vi "Test Data Graph01.vi"() -> ()   [LabVIEW 2020]
uses:
  <vilib>/measure/NI_MABase.lvlib
panel:
  in  "文件路径":path=path "C:/Users/26832/Desktop/20230719_134206.tdms"
  in  "Load":bool
  out "XY":cluster{timestamp[], dbl[]}[](graph)
  in  "P1":dbl(slide) scale=3772590125.497653..3772664225.497653 scale format="%<%m/%d %H:%M:%S>T"
  in  "P2":dbl(slide) scale=3772590125.497653..3772664225.497653 scale format="%<%m/%d %H:%M:%S>T"
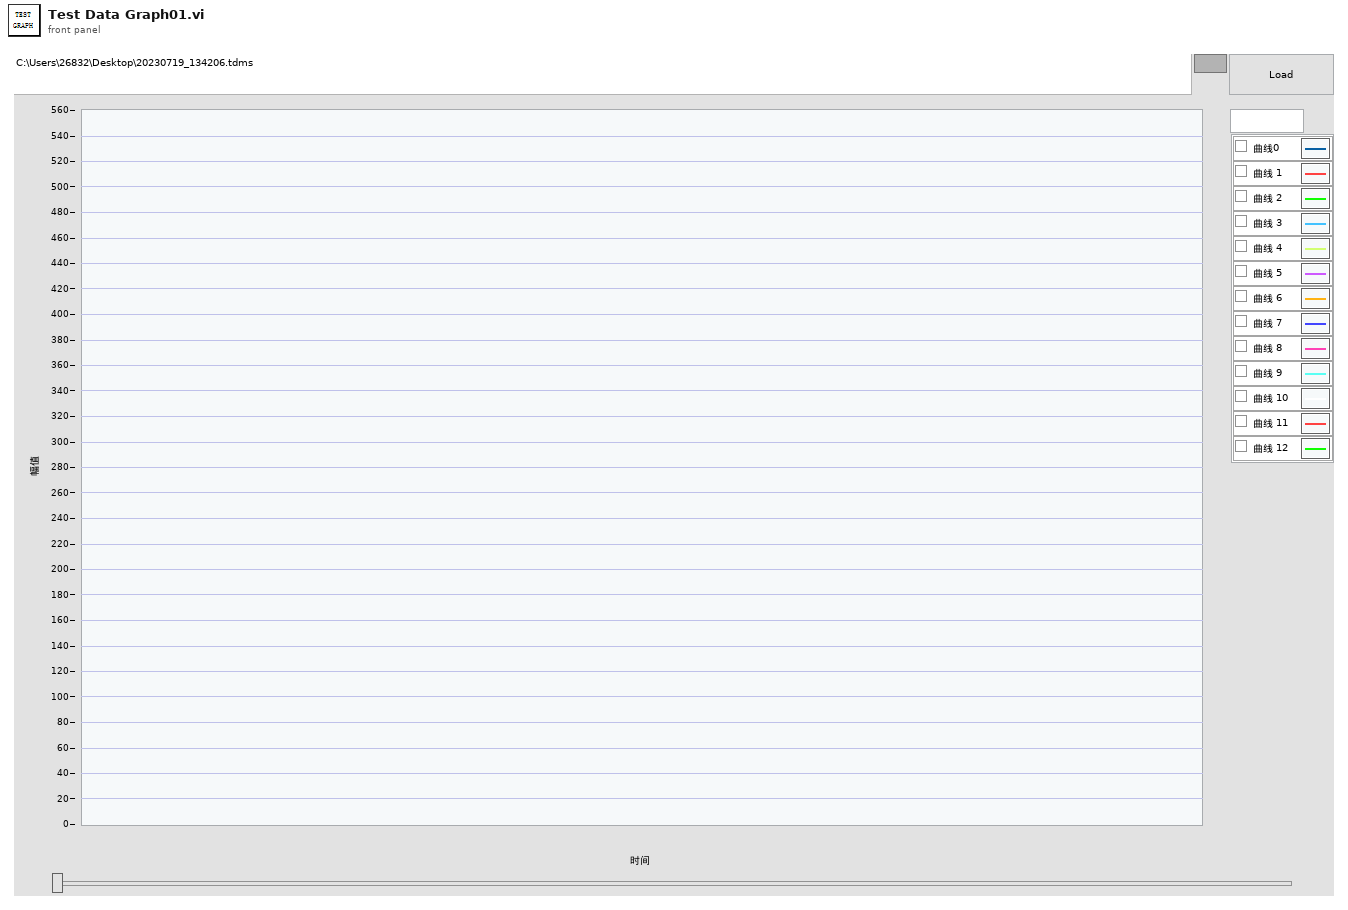
[diagram p1: front panel]
types:
  T1 = cluster{"XY":refnum<vi>, "Maxpoint":i32, "P1":refnum<vi>, "P2":refnum<vi>, "Range":cluster{"IStart":dbl, "CRange":dbl, "IRange":dbl, "CStart":dbl, "Stop":dbl}, "Wave":cluster{"Init":waveform(dbl), "Current":waveform(dbl)}}
  T2 = typedef "LVRangeTypeDef.ctl" = cluster{"Minimum":dbl, "Maximum":dbl, "Increment":dbl, "Minor Increment":dbl, "Start":dbl}
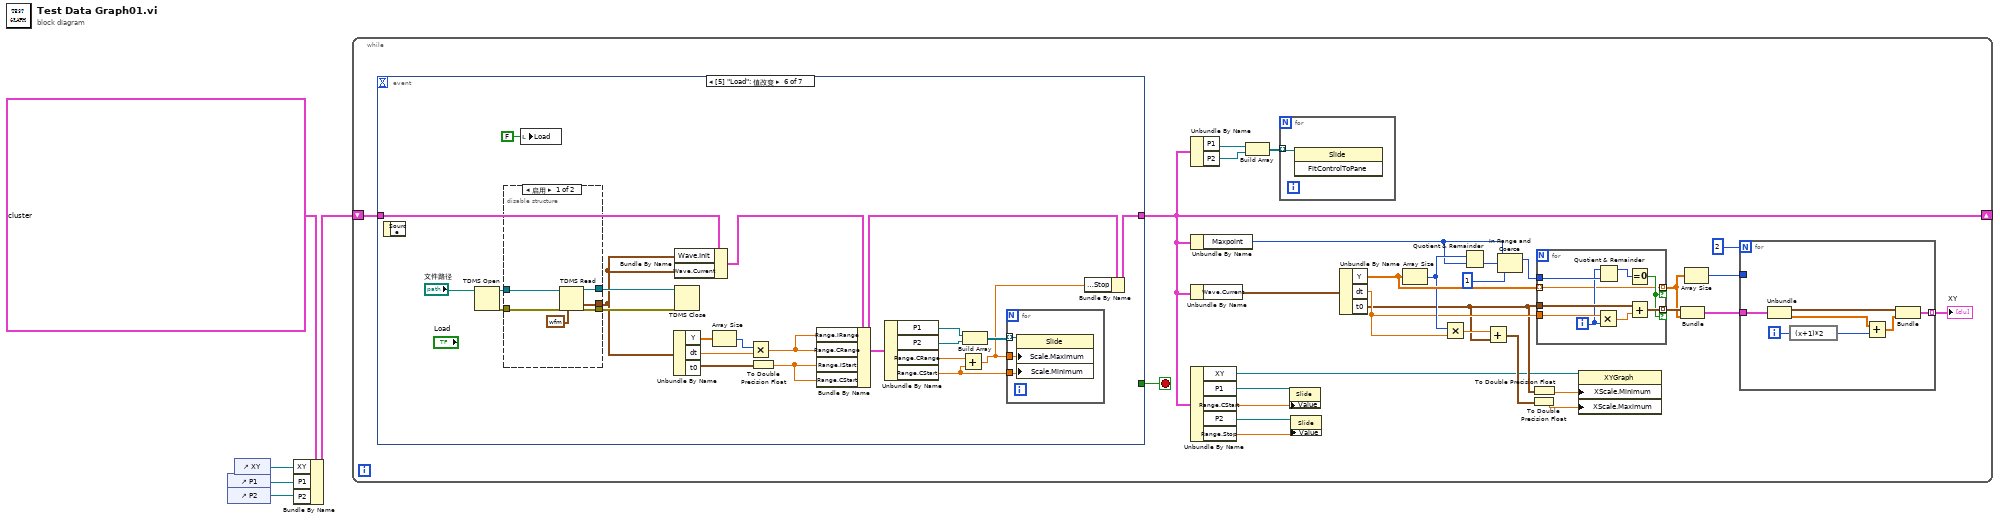
[diagram p0: block diagram]
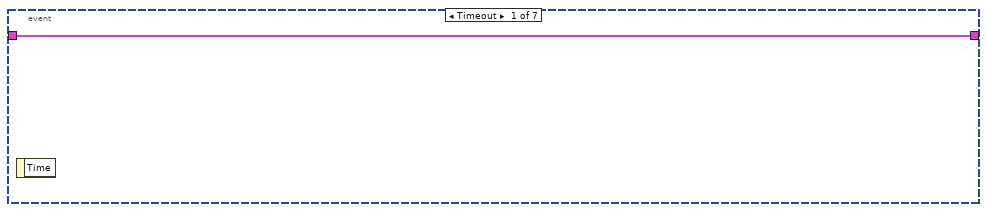
[diagram p2: hidden frame]
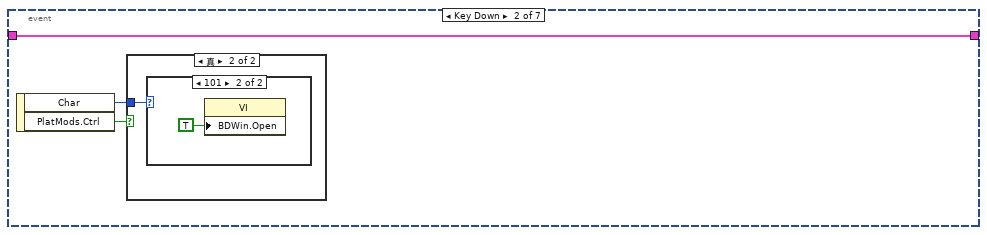
[diagram p3: hidden frame]
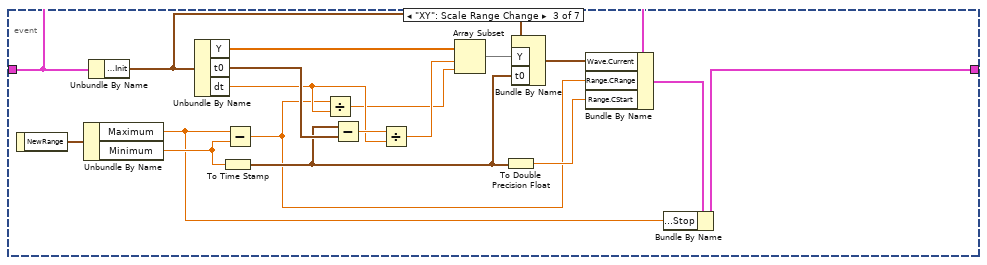
[diagram p6: hidden frame]
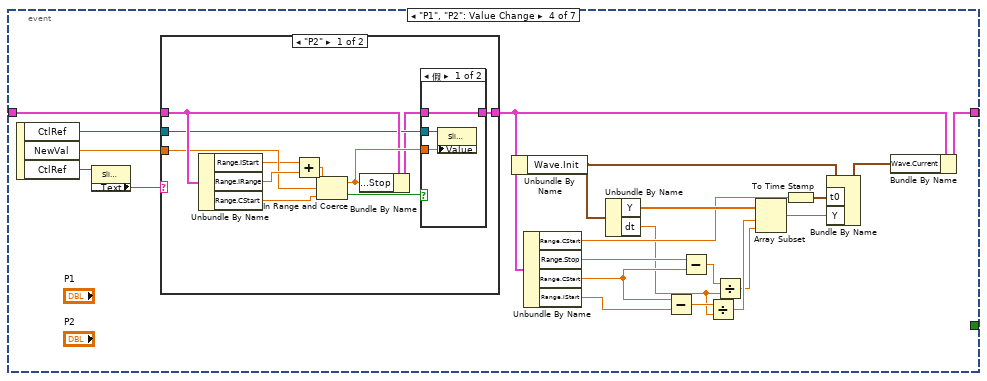
[diagram p7: hidden frame]
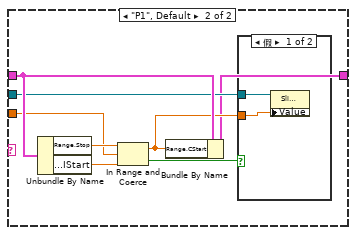
[diagram p9: hidden frame]
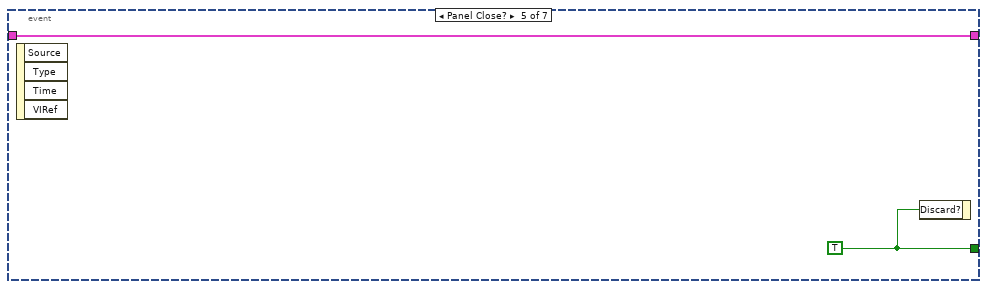
[diagram p11: hidden frame]
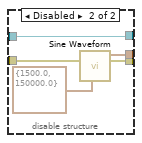
[diagram p12: hidden frame]
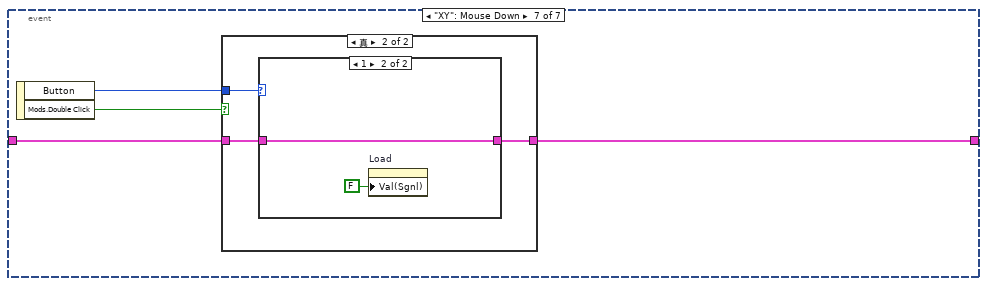
[diagram p13: hidden frame]
diagram:
  n1 = control-ref of="P1"() -> (w2:refnum<vi>)
  n2 = control-ref of="P2"() -> (w1:refnum<vi>)
  n3 = control-ref of="XY"() -> (w3:refnum<vi>)
  n4 = Bundle By Name(cluster=T1 {"XY"=refnum, "Maxpoint"=5000, "P1"=refnum, "P2"=refnum, "Range"={"IStart"=0.0, "CRange"=0.0, "IRange"=0.0, "CStart"=0.0, "Stop"=0.0}, "Wave"={"Init"={"t0"=timestamp(0 s since 1904-01-01), "dt"=1.0, "Y"=[]}, "Current"={"t0"=timestamp(0 s since 1904-01-01), "dt"=1.0, "Y"=[]}}}, "XY"=w3, "P1"=w2, "P2"=w1) -> (w4:T1)
  n5 = while {
    shift-right: [w9] -> _
    shift-left: w4 -> [w34]
    stop <- w35 stop-if-true
    n6 = event shown="[5] \"Load\": 值改变" {
      selector: _ -> [_ _ _ _ _ _ _]
      dyn-events: _ -> [_ _ _ _ _ _ _]
      timeout: _ -> [_ _ _ _ _ _ _]
      tunnel: [_ _ _ _ w124 _ _] -> w35
      tunnel: [w53 w54 w60 w95 w123 w128 w161] -> w9
      tunnel: w34 -> [w53 w54 w67 w97 w123 w142 w162]
      event Timeout {
        n7 = event-data() -> ()  [unwired: 1 in, 1 out]
      }
      event Key Down {
        n8 = event-data() -> ("Char"=w56:i16, "PlatMods.Ctrl"=w55:bool)  [unwired: 1 in]
        n9 = case shown="真" w55 {
          tunnel: w56 -> [_ w57]
          frame False {
          }
          frame True {
            n10 = case shown="101" w57 {
              frame 0, Default {
              }
              frame 101 {
                n11 = property class="VI"("BDWin.Open"=TRUE ("程序框图窗口:打开")) -> ()  [unwired: 2 in, 2 out]
              }
            }
          }
        }
      }
      event "XY": Scale Range Change {
        n12 = event-data() -> ("NewRange"=w76:T2)  [unwired: 1 in]
        n13 = Unbundle By Name(w76) -> ("Maximum"=w59:dbl, "Minimum"=w74:dbl)
        n14 = Unbundle By Name(w67) -> ("Wave.Init"=w66:waveform(dbl))
        n15 = Unbundle By Name(w66) -> ("Y"=w73:dbl[], "t0"=w75:timestamp, "dt"=w70:dbl)
        n16 = To Time Stamp(1:w74) -> (0:w63:timestamp)
        n17 = Subtract(x=w59, y=w74) -> (x-y=w61:dbl)
        n18 = Divide(x=w61, y=w70) -> (x/y=w68:dbl)
        n19 = Subtract(x=w63, y=w75) -> (x-y=w71:dbl)
        n20 = Divide(x=w71, y=w70) -> (x/y=w69:dbl)
        n21 = Array Subset(array=w73, index=w69, length=w68) -> (w72:dbl[])
        n22 = To Double Precision Float(number=w63) -> (double precision float=w62:dbl)
        n23 = Bundle By Name(cluster=w66, "Y"=w72, "t0"=w63) -> (w64:waveform(dbl))
        n24 = Bundle By Name(cluster=w67, "Wave.Current"=w64, "Range.CRange"=w61, "Range.CStart"=w62) -> (w65:T1)
        n25 = Bundle By Name(cluster=w65, "Range.Stop"=w59) -> (w60:T1)
      }
      event "P1", "P2": Value Change {
        n26 = event-data() -> ("CtlRef"=w79:refnum<vi>, "NewVal"=w96:dbl, "CtlRef"=w81:refnum<vi>)  [unwired: 1 in]
        n27 = property class="Slide (严格)"(reference=w81) -> ("Label.Text"=w80:string)  [unwired: 1 in, 2 out]
        n28 = case shown="\"P2\"" w80 {
          tunnel: w97 -> [w103 w120]
          tunnel: w96 -> [w101 w118]
          tunnel: w79 -> [w102 w116]
          tunnel: [w104 w113] -> w94
          frame "P2" {
            n29 = Unbundle By Name(w103) -> ("Range.IStart"=w99:dbl, "Range.IRange"=w106:dbl, "Range.CStart"=w98:dbl)
            n30 = Add(x=w99, y=w106) -> (x+y=w105:dbl)
            n31 = In Range and Coerce(upper limit=w105, x=w101, lower limit=w98) -> (coerced(x)=w108:dbl, In Range?=w107:bool)
            n32 = Bundle By Name(cluster=w103, "Range.Stop"=w108) -> (w100:T1)
            n33 = case shown="假" w107 {
              tunnel: w100 -> [w110 w112]
              tunnel: w108 -> [w111 _]
              tunnel: [w110 w112] -> w104
              tunnel: w102 -> [w109 _]
              frame False {
                n34 = property class="Slide (严格)"(reference=w109, "Value"=w111) -> ()  [unwired: 1 in, 2 out]
              }
              frame True {
              }
            }
          }
          frame "P1", Default {
            n35 = Unbundle By Name(w120) -> ("Range.Stop"=w119:dbl, "Range.IStart"=w117:dbl)
            n36 = In Range and Coerce(upper limit=w119, x=w118, lower limit=w117) -> (coerced(x)=w115:dbl, In Range?=w114:bool)
            n37 = Bundle By Name(cluster=w120, "Range.CStart"=w115) -> (w113:T1)
            n38 = case shown="假" w114 {
              tunnel: w116 -> [w122 _]
              tunnel: w115 -> [w121 _]
              frame False {
                n39 = property class="Slide (严格)"(reference=w122, "Value"=w121) -> ()  [unwired: 1 in, 2 out]
              }
              frame True {
              }
            }
          }
        }
        n40 = Unbundle By Name(w94) -> ("Wave.Init"=w90:waveform(dbl))
        n41 = Unbundle By Name(w94) -> ("Range.CStart"=w82:dbl, "Range.Stop"=w91:dbl, "Range.CStart"=w78:dbl, "Range.IStart"=w87:dbl)
        n42 = Unbundle By Name(w90) -> ("Y"=w88:dbl[], "dt"=w77:dbl)
        n43 = Subtract(x=w78, y=w87) -> (x-y=w86:dbl)
        n44 = Subtract(x=w91, y=w78) -> (x-y=w89:dbl)
        n45 = Divide(x=w86, y=w77) -> (x/y=w84:dbl)
        n46 = Divide(x=w89, y=w77) -> (x/y=w83:dbl)
        n47 = Array Subset(array=w88, index=w84, length=w83) -> (w85:dbl[])
        n48 = To Time Stamp(1:w82) -> (0:w93:timestamp)
        n49 = Bundle By Name(cluster=w90, "t0"=w93, "Y"=w85) -> (w92:waveform(dbl))
        n50 = Bundle By Name(cluster=w94, "Wave.Current"=w92) -> (w95:T1)
      }
      event Panel Close? {
        w124 = TRUE ("放弃？")
        n51 = event-data() -> ()  [unwired: 1 in, 4 out]
        n52 = event-data("Discard?"=w124) -> ()  [unwired: 1 in, 1 out]
      }
      event "Load": Value Change {
        n53 = event-data() -> ()  [unwired: 1 in, 1 out]
        n54 = TDMS Open(11:"文件路径") -> (0:w144:errorcluster, 3:w143:refnum<k34>)  [unwired: 6 in]
        n55 = disable-structure shown="启用" {
          disable-tunnel: [w153 w156] -> w146
          disable-tunnel: [w152 w157] -> w145
          disable-tunnel: w144 -> [w151 w156]
          disable-tunnel: w143 -> [w150 w157]
          disable-tunnel: [w148 w154] -> w126
          frame Enabled {
            n56 = TDMS Read(0:w150, 11:w151, 12:waveform(dbl) {"t0"=timestamp(0 s since 1904-01-01), "dt"=1.0, "Y"=[]} ("数据")) -> (4:w152:refnum<k34>, 10:w148:waveform(dbl), 15:w153:errorcluster)  [unwired: 5 in, 3 out]
          }
          frame Disabled {
            n57 = call <vilib>:"Sine Waveform.vi"("sampling info"=cluster{"Fs":dbl, "#s":dbl} {"Fs"=1500.0, "#s"=150000.0}) -> ("signal out"=w154:waveform(dbl))  [unwired: 9 in, 1 out]
          }
        }
        n58 = local write "Load"(FALSE ("Load")) -> ()
        n59 = Unbundle By Name(w126) -> ("Y"=w138:dbl[], "dt"=w139:dbl, "t0"=w140:timestamp)
        n60 = Bundle By Name(cluster=w142, "Wave.Init"=w126, "Wave.Current"=w126) -> (w141:T1)
        n61 = TDMS Close(8:w146, 11:w145) -> ()  [unwired: 2 out]
        n62 = Array Size(array=w138) -> (size(s)=w137:i32)
        n63 = Multiply(x=w137, y=w139) -> (x*y=w136:dbl)
        n64 = To Double Precision Float(number=w140) -> (double precision float=w130:dbl)
        n65 = Bundle By Name(cluster=w141, "Range.IRange"=w136, "Range.CRange"=w136, "Range.IStart"=w130, "Range.CStart"=w130) -> (w131:T1)
        n66 = Unbundle By Name(w131) -> ("P1"=w134:refnum<vi>, "P2"=w133:refnum<vi>, "Range.CRange"=w132:dbl, "Range.CStart"=w129:dbl)
        n67 = Add(x=w132, y=w129) -> (x+y=w127:dbl)
        n68 = Build Array(w134, w133) -> (w135:refnum<vi>[])
        n69 = for {
          tunnel: w135 -> [w160] mode=indexing
          tunnel: w127 -> [w159]
          tunnel: w129 -> [w158]
          n70 = property class="Slide"(reference=w160, "Scale.Maximum"=w159, "Scale.Minimum"=w158) -> ()  [unwired: 1 in, 2 out]
        }
        n71 = Bundle By Name(cluster=w131, "Range.Stop"=w127) -> (w128:T1)
      }
      event "XY": Mouse Down {
        n72 = event-data() -> ("Button"=w163:u16, "Mods.Double Click"=w164:bool)  [unwired: 1 in]
        n73 = case shown="真" w164 {
          tunnel: w163 -> [_ w168]
          tunnel: [w165 w167] -> w161
          tunnel: w162 -> [w165 w166]
          frame False {
          }
          frame True {
            n74 = case shown="1" w168 {
              tunnel: [w169 w171] -> w167
              tunnel: w166 -> [w169 w171]
              frame 0, Default {
              }
              frame 1 {
                n75 = property on="Load" class="Bool (严格)"("Val(Sgnl)"=FALSE ("值(信号)")) -> ()  [unwired: 2 in, 2 out]
              }
            }
          }
        }
      }
    }
    n76 = Unbundle By Name(w9) -> ("P1"=w10:refnum<vi>, "P2"=w11:refnum<vi>)
    n77 = Unbundle By Name(w9) -> ("Maxpoint"=w17:i32)
    n78 = Unbundle By Name(w9) -> ("Wave.Current"=w20:waveform(dbl))
    n79 = Unbundle By Name(w9) -> ("XY"=w16:refnum<vi>, "P1"=w15:refnum<vi>, "Range.CStart"=w13:dbl, "P2"=w14:refnum<vi>, "Range.Stop"=w8:dbl)
    n80 = Build Array(w10, w11) -> (w12:refnum<vi>[])
    n81 = for {
      tunnel: w12 -> [w36] mode=indexing
      n82 = invoke class="Slide" method="FitControlToPane"(reference=w36) -> ()  [unwired: 2 in, 3 out]
    }
    n83 = property class="Slide"(reference=w15, "Value"=w13) -> ()  [unwired: 1 in, 2 out]
    n84 = property class="Slide"(reference=w14, "Value"=w8) -> ()  [unwired: 1 in, 2 out]
    n85 = Unbundle By Name(w20) -> ("Y"=w32:dbl[], "dt"=w25:dbl, "t0"=w18:timestamp)
    n86 = Array Size(array=w32) -> (size(s)=w26:i32)
    n87 = Multiply(x=w26, y=w25) -> (x*y=w24:dbl)
    n88 = Quotient & Remainder(x=w26, y=w17) -> (floor(x/y)=w28:i32)  [unwired: 1 out]
    n89 = Add(x=w24, y=w18) -> (x+y=w22:timestamp)
    n90 = In Range and Coerce(upper limit=w17, x=w28, lower limit=1 ("下限")) -> (coerced(x)=w27:i32)  [unwired: 1 out]
    n91 = To Double Precision Float(number=w22) -> (double precision float=w21:dbl)
    n92 = To Double Precision Float(number=w18) -> (double precision float=w23:dbl)
    n93 = for {
      tunnel: w32 -> [w44] mode=indexing
      tunnel: w18 -> [w52]
      tunnel: w25 -> [w51]
      tunnel: [w49] -> w31 mode=indexing if=w48
      tunnel: [w44] -> w7 mode=indexing if=w48
      tunnel: w27 -> [w46]
      i -> [w45]
      n94 = Multiply(x=w51, y=w45) -> (x*y=w50:dbl)
      n95 = Quotient & Remainder(x=w45, y=w46) -> (x-y*floor(x/y)=w47:i32)  [unwired: 1 out]
      n96 = Equal To 0?(x=w47) -> (x = 0?=w48:bool)
      n97 = Add(x=w52, y=w50) -> (x+y=w49:timestamp)
    }
    n98 = property on="属性节点" class="XYGraph"(reference=w16, "XScale.Minimum"=w23, "XScale.Maximum"=w21) -> ()  [unwired: 1 in, 2 out]
    n99 = Bundle(w31, w7) -> (w33:cluster{timestamp[], dbl[]})  [unwired: 1 in]
    n100 = Array Size(array=w7) -> (size(s)=w6:i32)
    n101 = for {
      N: 2 -> [_]
      tunnel: w33 -> [w43]
      tunnel: [w37] -> w19 mode=indexing
      tunnel: w6 -> [_]
      i -> [w41]
      n102 = Unbundle(w43) -> (w39:timestamp[], w40:dbl[])
      n103 = expression code="(x+1)*2"(w41) -> (w42:i32)
      n104 = Add(x=w40, y=w42) -> (x+y=w38:dbl[])
      n105 = Bundle(w39, w38) -> (w37:cluster{timestamp[], dbl[]})  [unwired: 1 in]
    }
    "XY" <- w19
  }
